vi "Modify_Power_ElectrodesDlg.vi"(6 "error in":errorcluster, 8 "一行记录":string[](array[string])) -> (0 "error out":errorcluster)   [LabVIEW 2014, in "PowerElectrodes.lvlib"]
uses:
  PowerElectrodes.lvlib
  DataBase/DataBase.lvlib
  DetectElecrodes/DetectElectros.lvlib
panel:
  out "结果字符串":string
  in  "继电器极性":enum16{"负", "正", "    "}(ring)
  out "区域名称":string
  in  "确定按钮":bool
  in  "取消按钮":bool
  in  "继电器名称":string
  in  "电极描述":string
  in  "电极位置":string
  in  "坐标Z":string
  in  "坐标Y":string
  in  "坐标X":string
  in  "电极名称":string
  in  "区域名称":u16(ring) items=["1区", "2区"]
  in  "OK":bool
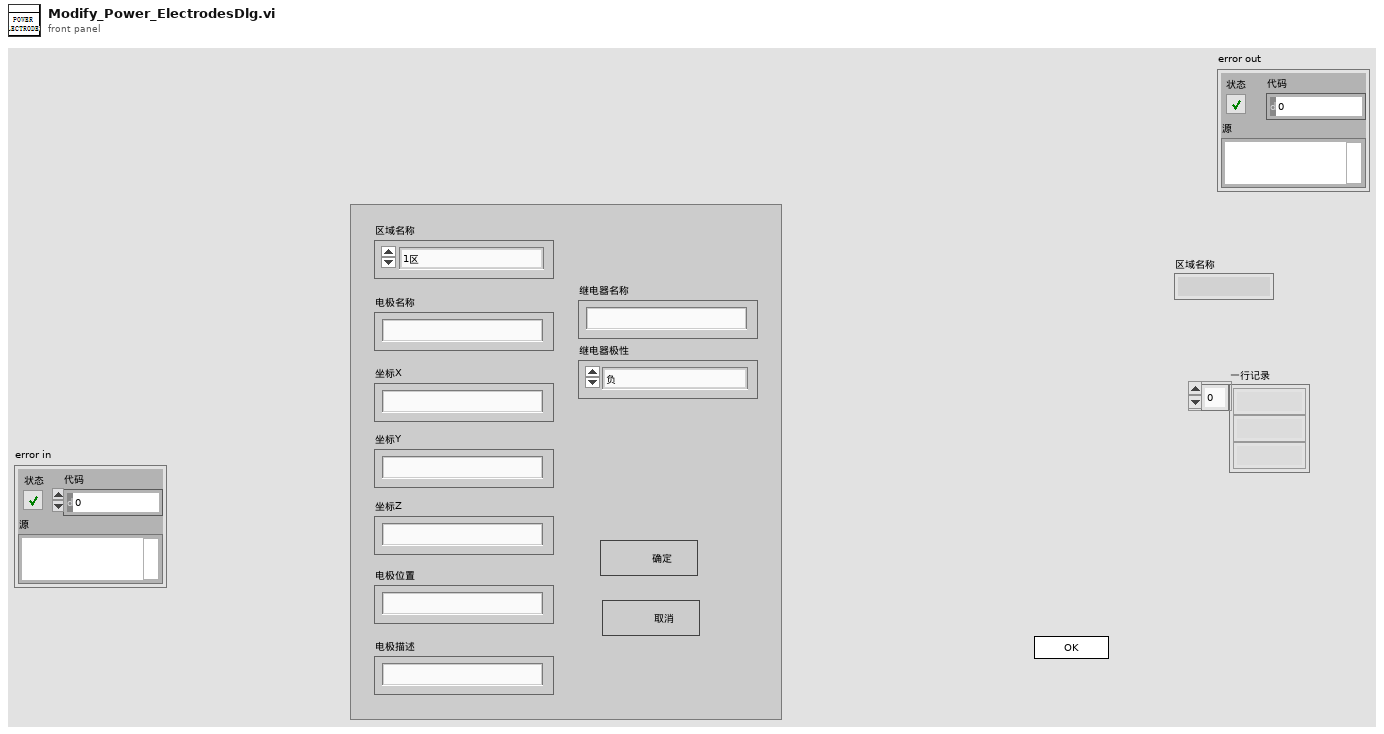
[diagram p1: front panel]
types:
  T1 = enum32{"invalid app kind", "Development System", "Run Time System", "Student Edition", "Embedded LabVIEW", "Evaluation", "Custom"}
  T2 = enum32{"Invalid", "Standard", "Closed", "Hidden", "Minimized", "Maximized"}
  T3 = cluster{"Core":cluster{"Current VI Reference":refnum<vi>, "Close Panel on Exit?":bool}, "Your Boolean data":bool, "Your string data":string, "AreaName":string[], "DataP":cluster{i32, "电极名称":string, "区域名称":string, "坐标X":string, "坐标Y":string, "坐标Z":string, "电极位置":string, "继电器名称":string, "继电器极性":string, "电极描述":string}, "一行记录D":string[], "power_id":string}
  T4 = cluster{i32, "电极名称":string, "区域名称":string, "坐标X":string, "坐标Y":string, "坐标Z":string, "电极位置":string, "继电器名称":string, "继电器极性":string, "电极描述":string}
  T5 = cluster{"Current VI Reference":refnum<vi>, "Close Panel on Exit?":bool}
  T6 = cluster{i32, "电极名称":string, "区域名称":string, "坐标X":string, "坐标Y":string, "坐标Z":string, "电极位置":string, "继电器名称":string, string, "电极描述":string}
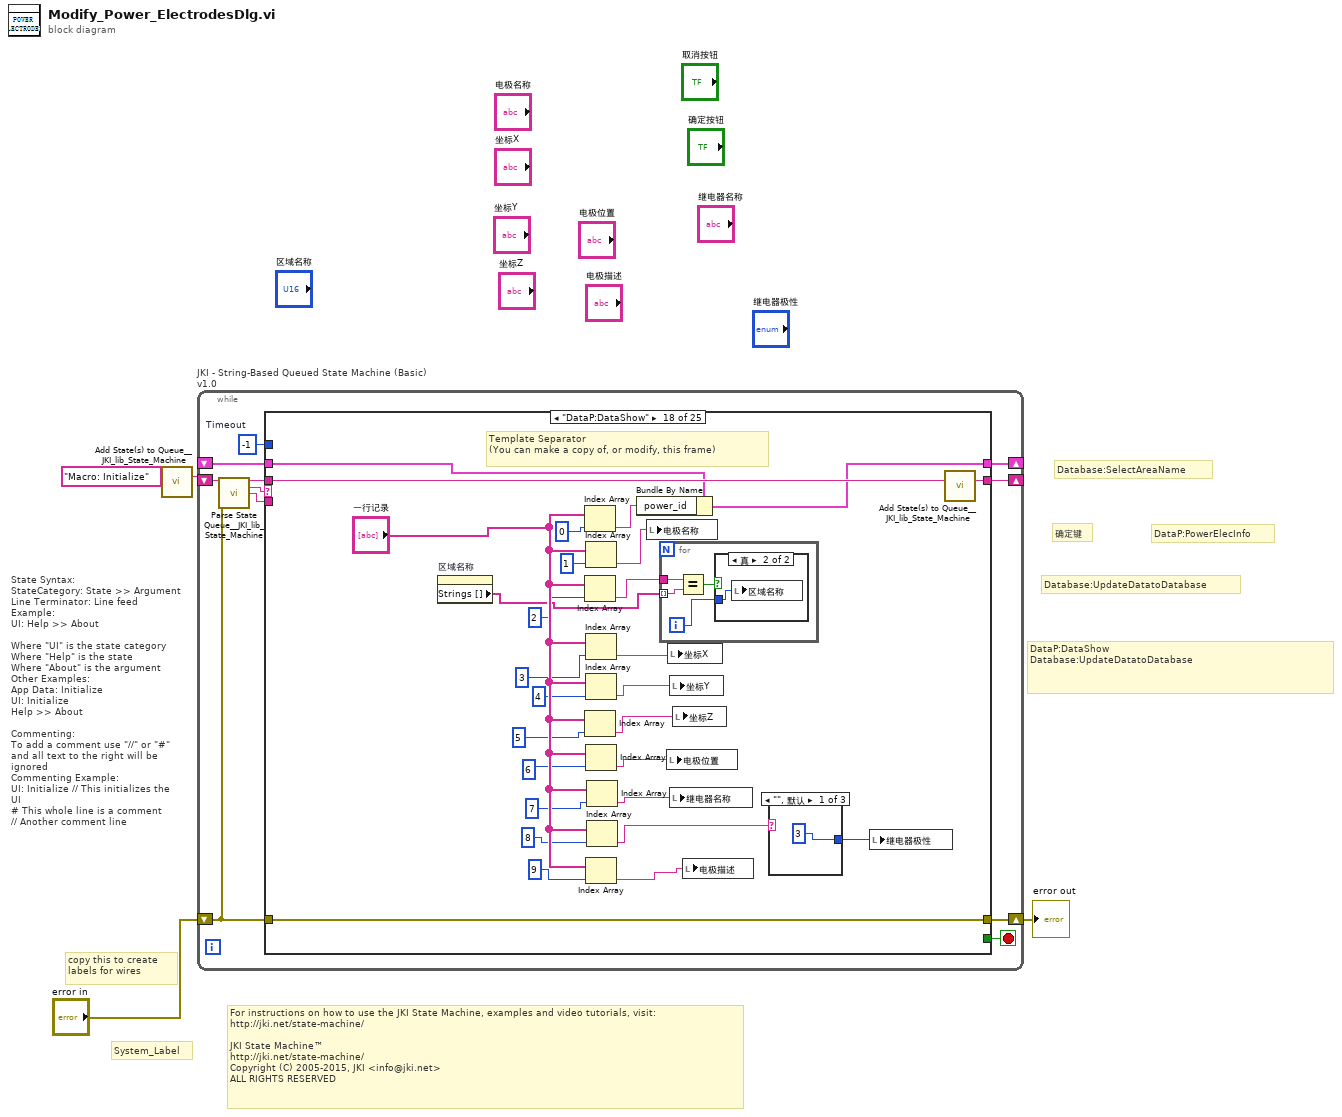
[diagram p0: block diagram]
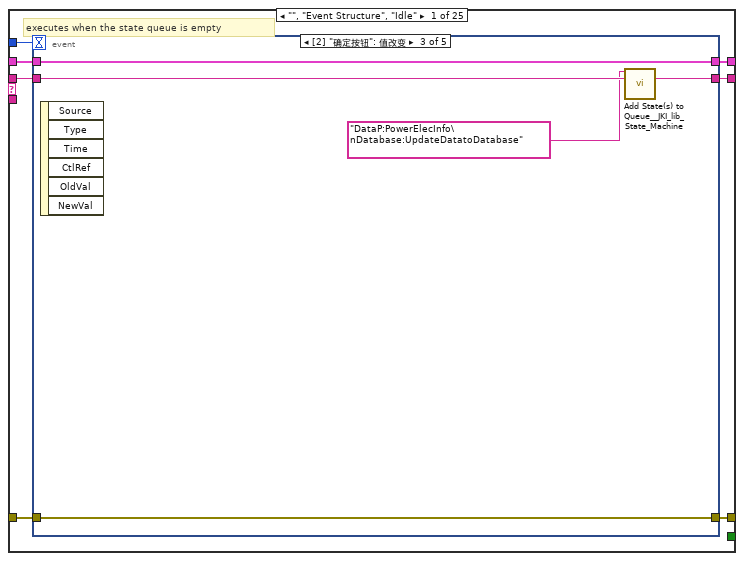
[diagram p2: hidden frame]
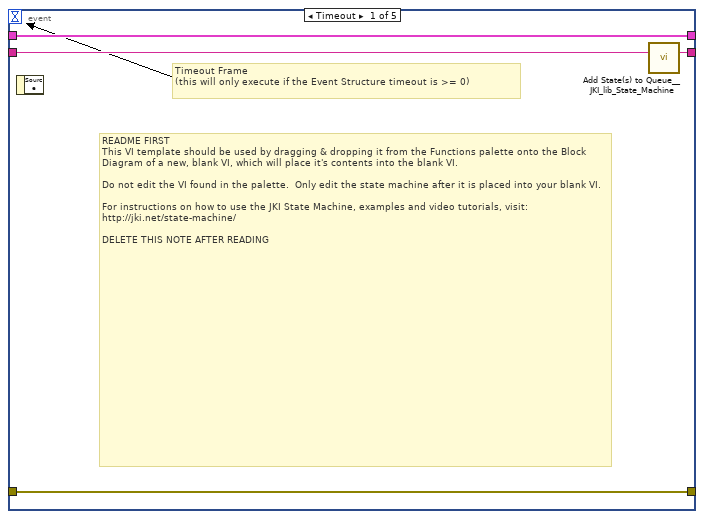
[diagram p3: hidden frame]
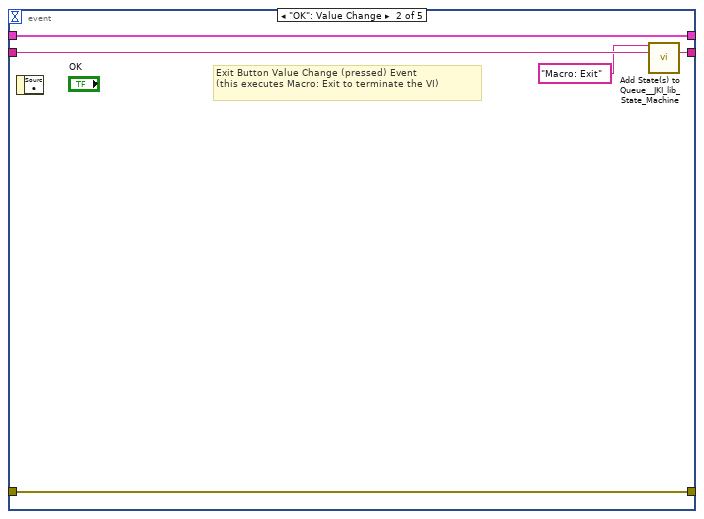
[diagram p4: hidden frame]
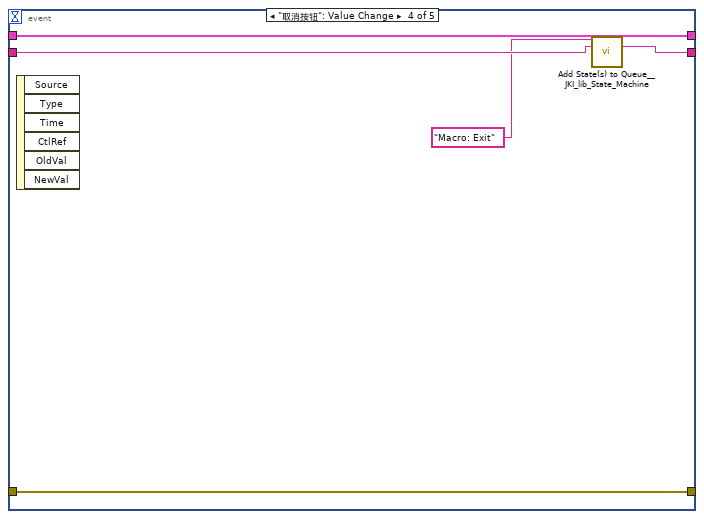
[diagram p5: hidden frame]
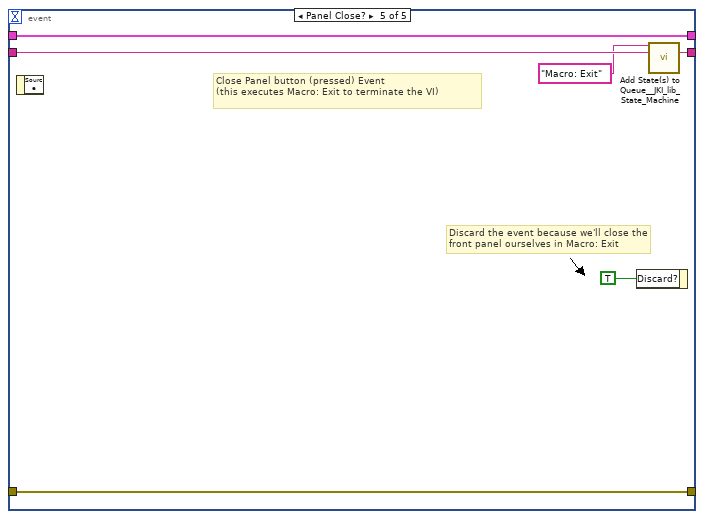
[diagram p6: hidden frame]
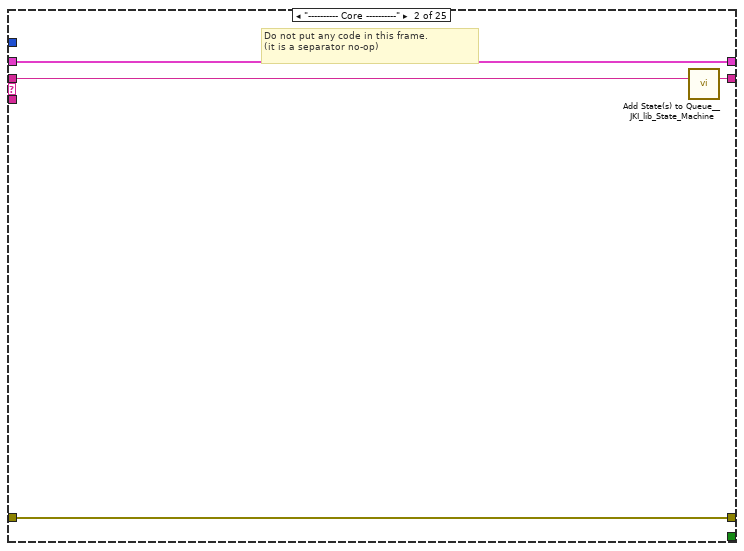
[diagram p7: hidden frame]
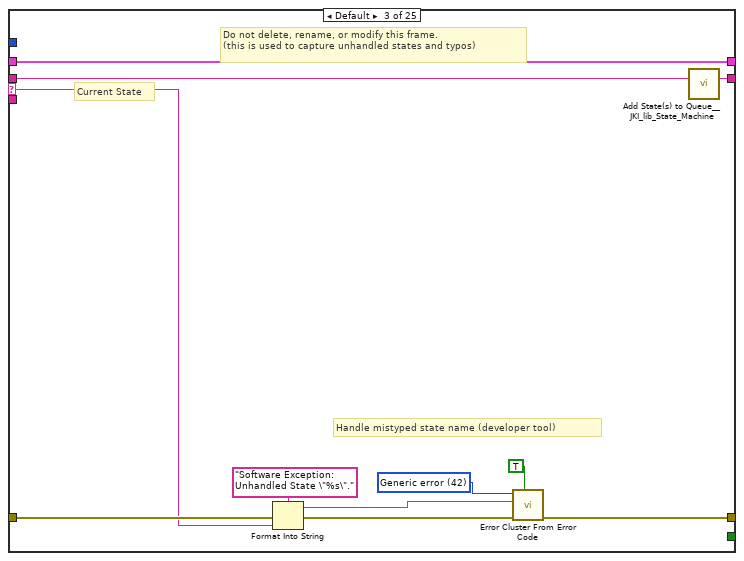
[diagram p8: hidden frame]
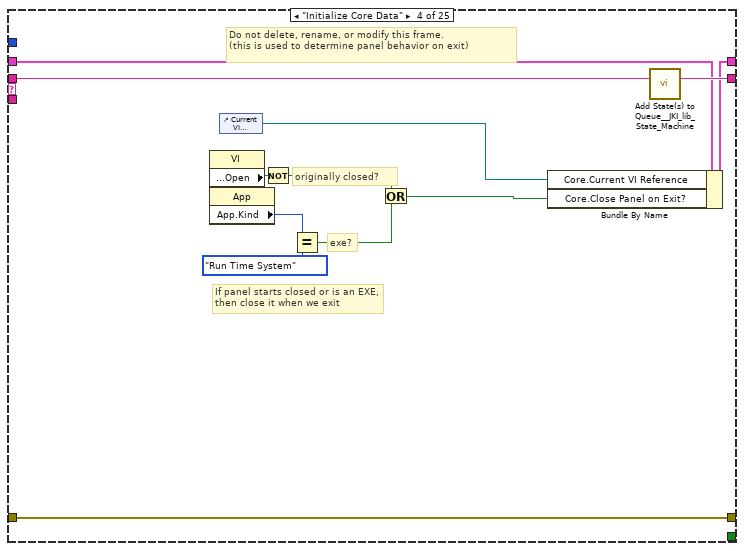
[diagram p9: hidden frame]
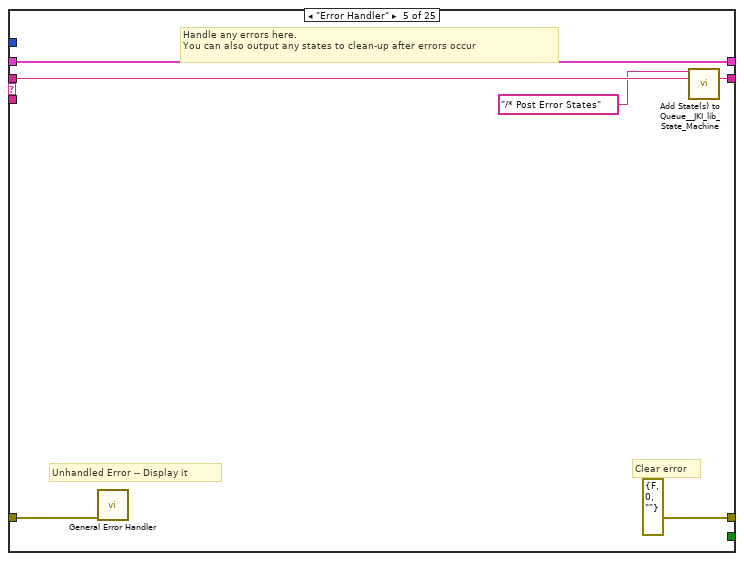
[diagram p10: hidden frame]
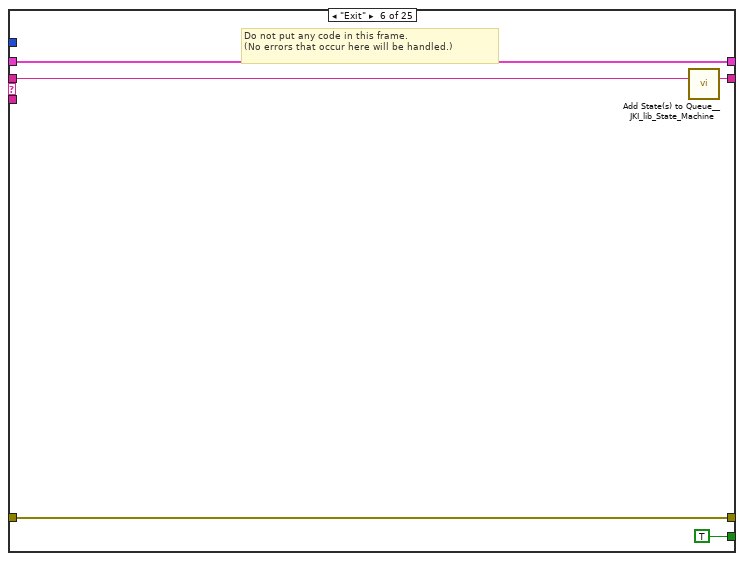
[diagram p11: hidden frame]
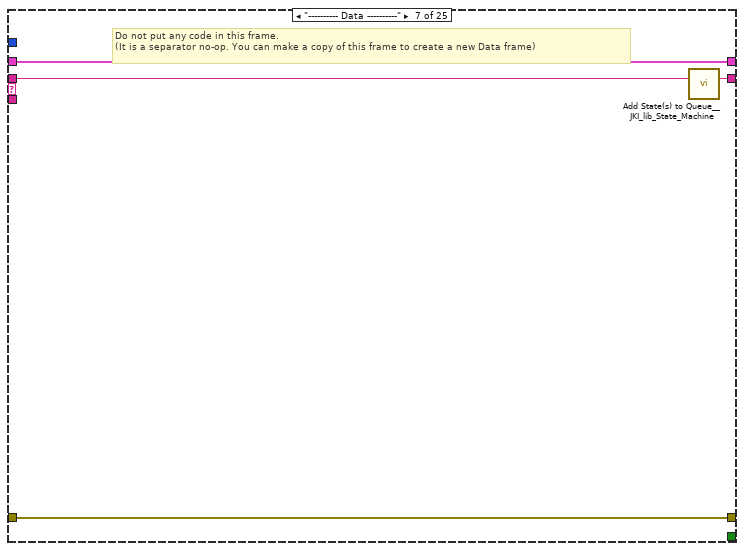
[diagram p12: hidden frame]
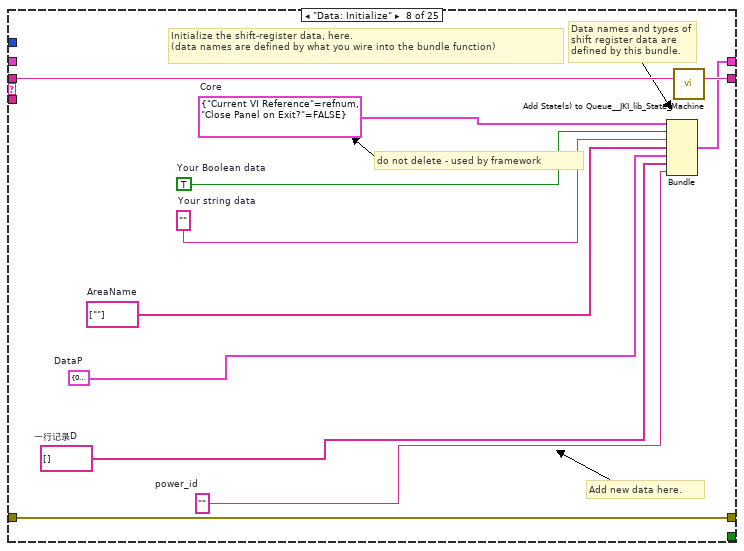
[diagram p13: hidden frame]
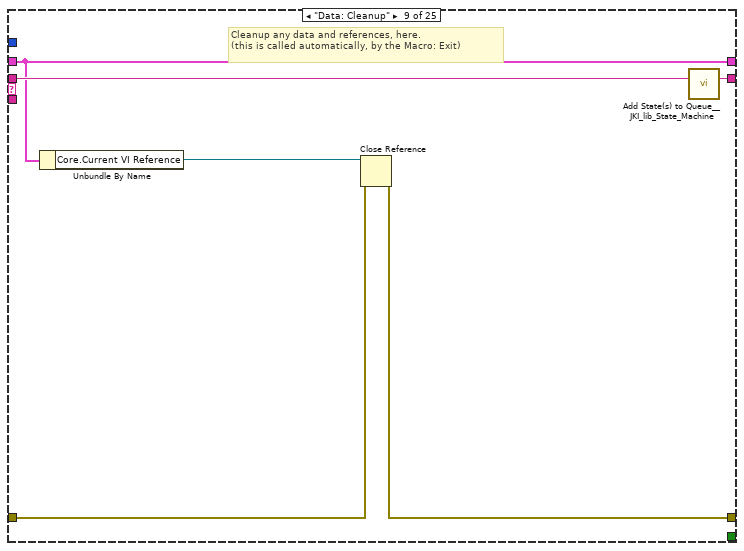
[diagram p14: hidden frame]
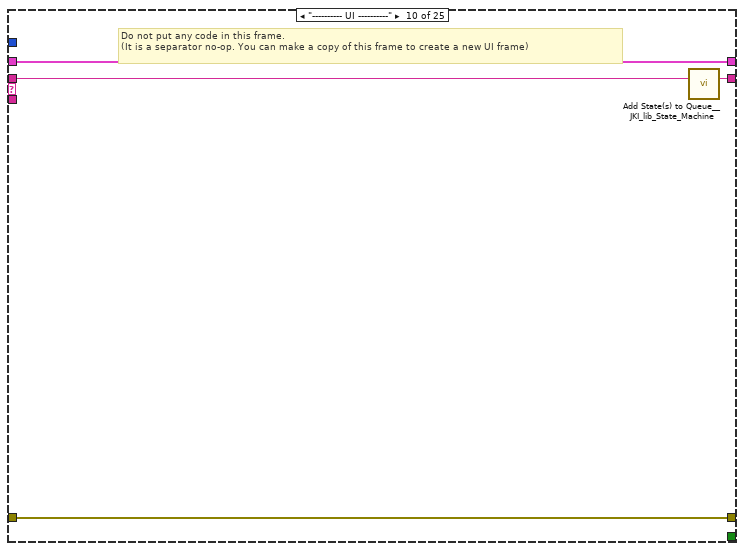
[diagram p15: hidden frame]
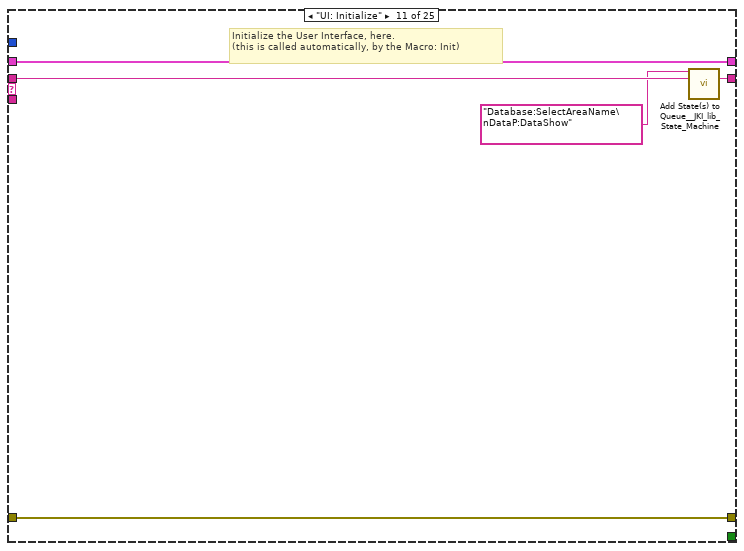
[diagram p16: hidden frame]
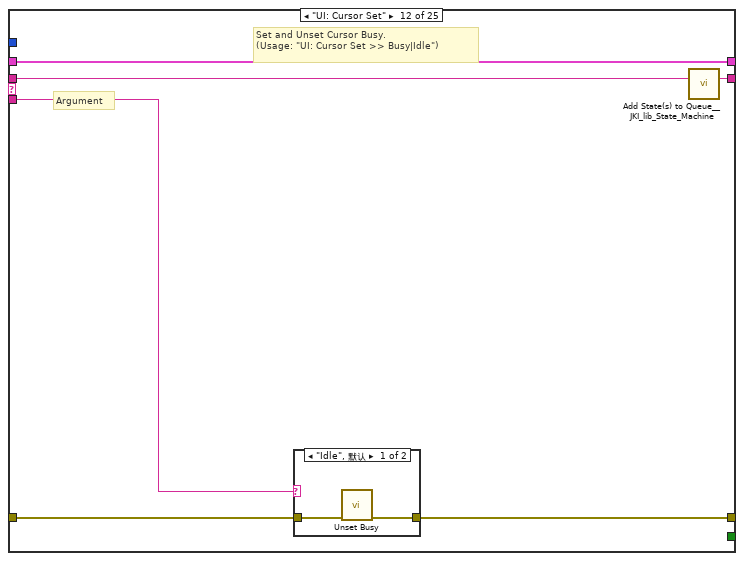
[diagram p17: hidden frame]
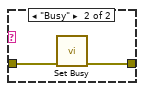
[diagram p18: hidden frame]
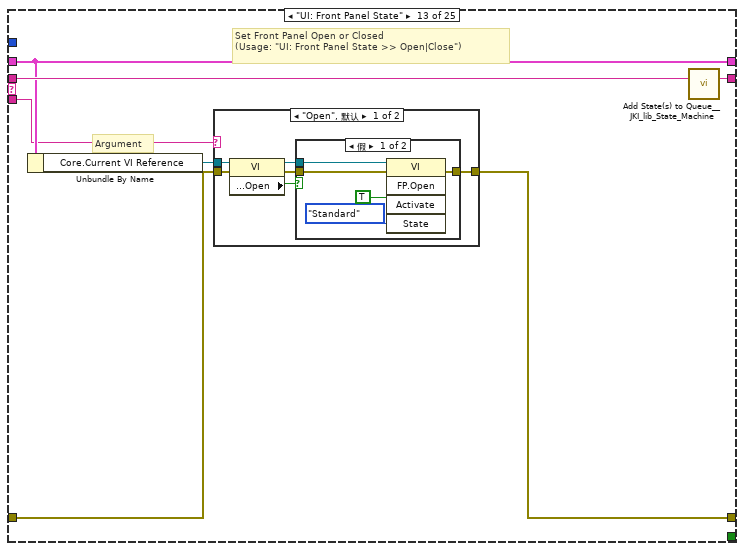
[diagram p19: hidden frame]
diagram:
  # "Database:UpdateDatatoDatabase"
  # "DataP:DataShow\nDatabase:UpdateDatatoDatabase"
  # "DataP:PowerElecInfo"
  # "确定键"
  # "Database:SelectAreaName"
  # "For instructions on how to use the JKI State Machine, examples and video tutorials, visit:\nhttp://jki.net/state-machine/\n\nJKI State Machine™\nhttp://jki.net/state-machine/\nCopyright (C) 2005-2015, JKI <info@jki.net>\nALL RIGHTS RESERVED"
  # "State Syntax:\nStateCategory: State >> Argument\nLine Terminator: Line feed\nExample:\nUI: Help >> About\n\nWhere \"UI\" is the state category\nWhere \"Help\" is the state\nWhere \"About\" is the argument\nOther Examples:\nApp Data: Initialize\nUI: Initialize\nHelp >> About\n\nCommenting:\nTo add a comment use \"//\" or \"#\" and all text to the right will be ignored\nCommenting Example:\nUI: Initialize // This initializes the UI\n# This whole line is a comment\n// Another comment line"
  # "copy this to create labels for wires"
  # "System_Label"
  n1 = call <vilib>:"Add State(s) to Queue__JKI_lib_State_Machine.vi"("State(s) in (\"\")"="Macro: Initialize") -> ("States Out"=w4:string)  [unwired: 14 in]
  n2 = while "JKI - String-Based Queued State Machine (Basic) v1.0" {
    shift-right: [w8] -> _
    shift-left: _ -> [w7]
    shift-right: [w11] -> w1
    shift-left: "error in" -> [w5]
    shift-right: [w10] -> _
    shift-left: w4 -> [w12]
    stop <- w9 stop-if-true
    w6 = -1  # Timeout
    n3 = call <vilib>:"Parse State Queue__JKI_lib_State_Machine.vi"("State Queue"=w12, "Error In (no error)"=w5) -> ("Remaining States"=w14:string, "Current State"=w15:string, "Arguments"=w13:string)  [unwired: 11 in]
    n4 = case shown="\"DataP:DataShow\"" w15 {
      selector: w15 -> [_ _ w52 _ _ _ _ _ _ _ _ _ _ _ _ _ _ _ _ _ _ _ _ _ _]
      tunnel: w14 -> [w22 w51 w56 w74 w80 w85 w89 w100 w106 w110 w115 w121 w132 w158 w163 w173 w177 w205 w234 w238 w260 w272 w276 w280 w284]
      tunnel: w13 -> [_ _ _ _ _ _ _ _ _ _ _ w116 w126 _ _ _ _ _ _ _ _ _ _ _ _]
      tunnel: w7 -> [w20 w48 w54 w65 w77 w83 w86 _ w101 w107 w113 w119 w128 w155 w160 w170 w174 w179 w220 w235 w257 w262 w273 w277 w281]
      tunnel: [w19 w49 w58 w71 errorcluster {"status"=FALSE, "code"=0, "source"=""} ("error out") w82 w87 w97 w102 w108 w111 w117 w129 w156 w161 w171 w175 w203 w232 w236 w240 w270 w274 w278 w282] -> w11
      tunnel: w5 -> [w18 w49 w57 w71 w76 w82 w87 w97 w103 w108 w111 w118 w130 w156 w161 w171 w175 w203 w232 w236 w239 w270 w274 w278 w282]
      tunnel: [w21 w50 w55 w73 w79 w84 w88 w99 w105 w109 w114 w120 w131 w157 w162 w172 w176 w204 w233 w237 w259 w271 w275 w279 w283] -> w10
      tunnel: [_ _ _ _ _ TRUE _ _ _ _ _ _ _ _ _ _ _ _ _ _ _ _ _ _ _] -> w9
      tunnel: [w17 w48 w54 w72 w77 w83 w86 w98 w101 w107 w113 w119 w128 w155 w160 w170 w174 w178 w219 w235 w257 w261 w273 w277 w281] -> w8
      tunnel: w6 -> [w16 _ _ _ _ _ _ _ _ _ _ _ _ _ _ _ _ _ _ _ _ _ _ _ _]
      frame "", "Event Structure", "Idle" {
        # "executes when the state queue is empty"
        n5 = event shown="[2] \"确定按钮\": 值改变" {
          selector: _ -> [_ _ _ _ _]
          dyn-events: _ -> [_ _ _ _ _]
          timeout: w16 -> [_ _ _ _ _]
          tunnel: w22 -> [w26 w31 w33 w39 w47]
          tunnel: [w25 w30 w34 w40 w46] -> w21
          tunnel: w20 -> [w23 w28 w36 w41 w44]
          tunnel: [w24 w29 w35 w37 w45] -> w19
          tunnel: w18 -> [w24 w29 w35 w37 w45]
          tunnel: [w23 w28 w36 w41 w44] -> w17
          event Timeout {
            # "README FIRST\nThis VI template should be used by dragging & dropping it from the Functions palette onto the Block Diagram of a new, blank VI, which will place it's contents into the blank VI.\n\nDo not edit the VI found in the palette.  Only edit the state machine after it is placed into your blank VI.\n\nFor instructions on how to use the JKI State Machine, examples and video tutorials, visit:\nhttp://jki.net/state-machine/\n\nDELETE THIS NOTE AFTER READING"
            # "Timeout Frame\n(this will only execute if the Event Structure timeout is >= 0)"
            n6 = event-data() -> ()  [unwired: 1 in, 1 out]
            n7 = call <vilib>:"Add State(s) to Queue__JKI_lib_State_Machine.vi"("State(s) in (\"\")"=w26) -> ("States Out"=w25:string)  [unwired: 14 in]
          }
          event "OK": Value Change {
            # "Exit Button Value Change (pressed) Event\n(this executes Macro: Exit to terminate the VI)"
            n8 = event-data() -> ()  [unwired: 1 in, 1 out]
            n9 = call <vilib>:"Add State(s) to Queue__JKI_lib_State_Machine.vi"("State(s) in Front (\"\")"="Macro: Exit", "State(s) in (\"\")"=w31) -> ("States Out"=w30:string)  [unwired: 13 in]
          }
          event "确定按钮": Value Change {
            n10 = event-data() -> ()  [unwired: 1 in, 6 out]
            n11 = call <vilib>:"Add State(s) to Queue__JKI_lib_State_Machine.vi"("State(s) in Front (\"\")"="DataP:PowerElecInfo\nDatabase:UpdateDatatoDatabase", "State(s) in (\"\")"=w33) -> ("States Out"=w34:string)  [unwired: 13 in]
          }
          event "取消按钮": Value Change {
            n12 = event-data() -> ()  [unwired: 1 in, 6 out]
            n13 = call <vilib>:"Add State(s) to Queue__JKI_lib_State_Machine.vi"("State(s) in Front (\"\")"="Macro: Exit", "State(s) in (\"\")"=w39) -> ("States Out"=w40:string)  [unwired: 13 in]
          }
          event Panel Close? {
            # "Discard the event because we'll close the front panel ourselves in Macro: Exit"
            # "Close Panel button (pressed) Event\n(this executes Macro: Exit to terminate the VI)"
            n14 = event-data() -> ()  [unwired: 1 in, 1 out]
            n15 = event-data("Discard?"=TRUE) -> ()  [unwired: 1 in, 1 out]
            n16 = call <vilib>:"Add State(s) to Queue__JKI_lib_State_Machine.vi"("State(s) in Front (\"\")"="Macro: Exit", "State(s) in (\"\")"=w47) -> ("States Out"=w46:string)  [unwired: 13 in]
          }
        }
      }
      frame "---------- Core ----------" {
        # "Do not put any code in this frame.\n(it is a separator no-op)"
        n17 = call <vilib>:"Add State(s) to Queue__JKI_lib_State_Machine.vi"("State(s) in (\"\")"=w51) -> ("States Out"=w50:string)  [unwired: 14 in]
      }
      frame Default {
        w61 = 42 items=["No error", "Argument error", "Memory is full", "Out of zone", "End of file", "File already open", "Generic file I/O error", "File not found", "File permission error", "Disk is full", "Duplicate path", "Too many files open", "System feature not enabled", "Resource file not found", "Cannot add resource", "Resource not found", "Image not found", "Image memory error", "Pen does not exist", "Config type invalid", "Config token not found", "Config parse error", "Config memory error", "Bad external code format", "Bad external code offset", "External code not present", "Null window", "Destroy window error", "Null menu", "Print aborted", "Bad print record", "Print driver error", "Windows error during printing", "Memory error during printing", "Print dialog error", "Generic print error", "Invalid device refnum", "Device not found", "Device parameter error", "Device unit error", "Cannot open device", "Device call aborted", "Generic error", "Cancelled by user", "Object ID too low", "Object ID too high", "Object not in heap", "Unknown heap", "Unknown object (invalid DefProc)", "Unknown object (DefProc not in table)", "Message out of range", "Invalid (null) method", "Unknown message", "Manager call not supported", "Bad address", "Network operation in progress", "Network operation timed out", "Connection is busy", "Network attribute not supported", "Network error", "Address in use", "System out of memory", "Connection aborted", "Connection refused", "Not connected", "Already connected", "Connection closed", "Initialization error (interapplication manager)", "Bad occurrence", "Wait on unbound occurrence handler", "Occurrence queue overflow", "Datalog type conflict", "Unused", "Unrecognized type (interapplication manager)", "Memory corrupt", "Failed to make temporary DLL", "Old CIN version", "Drag socket not found", "Failed to load drop-object", "Failed to register OLE object", "Failed to release OLE object", "Format specifier type mismatch", "Unknown format specifier", "Too few format specifiers", "Too many format specifiers", "Scan failed", "Newer CIN version", "Error converting to variant", "Runtime menu error", "Password tampered", "Variant attribute not found", "Incompatible variant data type", "Event data is not available", "Event Store is not present", "Occurrence is not found", "Event Queue is not created", "Event info is not available", "Refnum passed is NULL", "Error retrieving Class GUID", "Error retrieving CoClass GUID", "Error retrieving TypeLib GUID.", "Bad built application magic bytes.", "Specific driver is different from the specific driver associated with the Logical Name.", "There is no session opened to the class driver.", "Max Error", "MAX - Error with config objects", "MAX - Error loading configuration", "MAX - Group not supported"]
        # "Current State"
        # "Do not delete, rename, or modify this frame.\n(this is used to capture unhandled states and typos)"
        # "Handle mistyped state name (developer tool)"
        n18 = Format Into String(format string="Software Exception: Unhandled State \"%s\"." ("message"), error in=w57, w52) -> (resulting string=w60:string, error out=w59:errorcluster)  [unwired: 1 in]
        n19 = call <vilib>:"Error Cluster From Error Code.vi"("show call chain? (False)"=TRUE, "error in (no error)"=w59, "error message (\"\")"=w60, "error code (0)"=w61) -> ("error out"=w58:errorcluster)  [unwired: 5 in]
        n20 = call <vilib>:"Add State(s) to Queue__JKI_lib_State_Machine.vi"("State(s) in (\"\")"=w56) -> ("States Out"=w55:string)  [unwired: 14 in]
      }
      frame "Initialize Core Data" {
        # "Do not delete, rename, or modify this frame.\n(this is used to determine panel behavior on exit)"
        # "originally closed?"
        # "exe?"
        # "If panel starts closed or is an EXE, then close it when we exit"
        n21 = property class="VI"() -> ("Front Panel.Open"=w70:bool)  [unwired: 2 in, 2 out]
        n22 = property class="App"() -> ("App.Kind"=w69:T1)  [unwired: 2 in, 2 out]
        n23 = control-ref of="Current VI Reference"() -> (w63:refnum<vi>)
        n24 = Not(x=w70) -> (.not. x?=w67:bool)
        n25 = Equal?(x=w69, y=T1."Run Time System" ("Application:Kind")) -> (x = y?=w66:bool)
        n26 = Or(x=w67, y=w66) -> (x .or. y?=w64:bool)
        n27 = Bundle By Name(cluster=w65, "Core.Current VI Reference"=w63, "Core.Close Panel on Exit?"=w64) -> (w72:T3)
        n28 = call <vilib>:"Add State(s) to Queue__JKI_lib_State_Machine.vi"("State(s) in (\"\")"=w74) -> ("States Out"=w73:string)  [unwired: 14 in]
      }
      frame "Error Handler" {
        # "Unhandled Error -- Display it"
        # "Handle any errors here.\nYou can also output any states to clean-up after errors occur"
        # "Clear error"
        n29 = call <vilib>:"General Error Handler.vi"("error in (no error)"=w76) -> ()  [unwired: 10 in, 5 out]
        n30 = call <vilib>:"Add State(s) to Queue__JKI_lib_State_Machine.vi"("State(s) in Front (\"\")"="/* Post Error States", "State(s) in (\"\")"=w80) -> ("States Out"=w79:string)  [unwired: 13 in]
      }
      frame "Exit" {
        # "Do not put any code in this frame.\n(No errors that occur here will be handled.)"
        n31 = call <vilib>:"Add State(s) to Queue__JKI_lib_State_Machine.vi"("State(s) in (\"\")"=w85) -> ("States Out"=w84:string)  [unwired: 14 in]
      }
      frame "---------- Data ----------" {
        # "Do not put any code in this frame.\n(It is a separator no-op. You can make a copy of this frame to create a new Data frame)"
        n32 = call <vilib>:"Add State(s) to Queue__JKI_lib_State_Machine.vi"("State(s) in (\"\")"=w89) -> ("States Out"=w88:string)  [unwired: 14 in]
      }
      frame "Data: Initialize" {
        w90 = ""  # power_id
        w91 = string[] []  # 一行记录D
        w92 = T4 {0, "电极名称"="", "区域名称"="", "坐标X"="", "坐标Y"="", "坐标Z"="", "电极位置"="", "继电器名称"="", "继电器极性"="", "电极描述"=""}  # DataP
        w93 = string[] [""]  # AreaName
        w94 = T5 {"Current VI Reference"=refnum, "Close Panel on Exit?"=FALSE}  # Core
        w96 = TRUE  # Your Boolean data
        w95 = ""  # Your string data
        # "do not delete - used by framework"
        # "Add new data here."
        # "Data names and types of shift register data are defined by this bundle."
        # "Initialize the shift-register data, here.\n(data names are defined by what you wire into the bundle function)"
        n33 = Bundle("Core"=w94, "Your Boolean data"=w96, "Your string data"=w95, "AreaName"=w93, "DataP"=w92, "一行记录D"=w91, "power_id"=w90) -> (w98:T3)  [unwired: 1 in]
        n34 = call <vilib>:"Add State(s) to Queue__JKI_lib_State_Machine.vi"("State(s) in (\"\")"=w100) -> ("States Out"=w99:string)  [unwired: 14 in]
      }
      frame "Data: Cleanup" {
        # "Cleanup any data and references, here.\n(this is called automatically, by the Macro: Exit)"
        n35 = Unbundle By Name(w101) -> ("Core.Current VI Reference"=w104:refnum<vi>)
        n36 = Close Reference(reference=w104, error in (no error)=w103) -> (error out=w102:errorcluster)
        n37 = call <vilib>:"Add State(s) to Queue__JKI_lib_State_Machine.vi"("State(s) in (\"\")"=w106) -> ("States Out"=w105:string)  [unwired: 14 in]
      }
      frame "---------- UI ----------" {
        # "Do not put any code in this frame.\n(It is a separator no-op. You can make a copy of this frame to create a new UI frame)"
        n38 = call <vilib>:"Add State(s) to Queue__JKI_lib_State_Machine.vi"("State(s) in (\"\")"=w110) -> ("States Out"=w109:string)  [unwired: 14 in]
      }
      frame "UI: Initialize" {
        # "Initialize the User Interface, here.\n(this is called automatically, by the Macro: Init)"
        n39 = call <vilib>:"Add State(s) to Queue__JKI_lib_State_Machine.vi"("State(s) in Front (\"\")"="Database:SelectAreaName\nDataP:DataShow", "State(s) in (\"\")"=w115) -> ("States Out"=w114:string)  [unwired: 13 in]
      }
      frame "UI: Cursor Set" {
        # "Argument"
        # "Set and Unset Cursor Busy.\n(Usage: \"UI: Cursor Set >> Busy|Idle\")"
        n40 = case shown="\"Idle\", 默认" w116 {
          tunnel: w118 -> [w123 w125]
          tunnel: [w122 w124] -> w117
          frame "Idle", Default {
            n41 = call <vilib>:"Unset Busy.vi"("error in (no error)"=w123) -> ("error out"=w122:errorcluster)  [unwired: 10 in]
          }
          frame "Busy" {
            n42 = call <vilib>:"Set Busy.vi"("error in (no error)"=w125) -> ("error out"=w124:errorcluster)  [unwired: 9 in, 1 out]
          }
        }
        n43 = call <vilib>:"Add State(s) to Queue__JKI_lib_State_Machine.vi"("State(s) in (\"\")"=w121) -> ("States Out"=w120:string)  [unwired: 14 in]
      }
      frame "UI: Front Panel State" {
        # "Argument"
        # "Set Front Panel Open or Closed\n(Usage: \"UI: Front Panel State >> Open|Close\")"
        n44 = Unbundle By Name(w128) -> ("Core.Current VI Reference"=w127:refnum<vi>)
        n45 = case shown="\"Open\", 默认" w126 {
          tunnel: w130 -> [w136 w149]
          tunnel: [w138 w150] -> w129
          tunnel: w127 -> [w137 w147]
          frame "Open", Default {
            n46 = property class="VI"(reference=w137, error in=w136) -> (reference out=w134:refnum<vi>, error out=w135:errorcluster, "Front Panel.Open"=w133:bool)
            n47 = case shown="假" w133 {
              tunnel: [w141 w144] -> w138
              tunnel: w135 -> [w140 w144]
              tunnel: w134 -> [w139 _]
              frame False {
                n48 = invoke class="VI" method="FP.Open"(reference=w139, error in=w140, "Activate"=TRUE, "State"=T2."Standard") -> (error out=w141:errorcluster)  [unwired: 1 in, 4 out]
              }
              frame True {
              }
            }
          }
          frame "Close" {
            n49 = property class="VI"(reference=w147, error in=w149) -> (reference out=w146:refnum<vi>, error out=w148:errorcluster, "Front Panel.Open"=w145:bool)
            n50 = case shown="真" w145 {
              tunnel: [w151 w154] -> w150
              tunnel: w148 -> [w151 w153]
              tunnel: w146 -> [_ w152]
              frame False {
              }
              frame True {
                n51 = invoke class="VI" method="FP.Close"(reference=w152, error in=w153) -> (error out=w154:errorcluster)  [unwired: 1 in, 2 out]
              }
            }
          }
        }
        n52 = call <vilib>:"Add State(s) to Queue__JKI_lib_State_Machine.vi"("State(s) in (\"\")"=w132) -> ("States Out"=w131:string)  [unwired: 14 in]
      }
      frame "---------- Macro ----------" {
        # "Do not put any code in this frame.\n(It is a separator no-op. You can make a copy of this frame to create a new Macro frame)"
        n53 = call <vilib>:"Add State(s) to Queue__JKI_lib_State_Machine.vi"("State(s) in (\"\")"=w158) -> ("States Out"=w157:string)  [unwired: 14 in]
      }
      frame "Macro: Initialize" {
        w159 = "Data: Initialize\nInitialize Core Data\nUI: Initialize\nUI: Front Panel State >> Open"  # Data: Initialize Initialize Core Data UI: Initialize UI: Front Panel State >> Open
        # "Initialization Macro\n(This is called once, when the VI starts)"
        n54 = call <vilib>:"Add State(s) to Queue__JKI_lib_State_Machine.vi"("State(s) in Front (\"\")"=w159, "State(s) in (\"\")"=w163) -> ("States Out"=w162:string)  [unwired: 13 in]
      }
      frame "Macro: Exit" {
        # "Exit Macro\n(This is called once, when the VI exits)"
        n55 = Unbundle By Name(w170) -> ("Core.Close Panel on Exit?"=w169:bool)
        n56 = Select(t="UI: Front Panel State >> Close", s=w169, f="") -> (s? t:f=w166:string)
        n57 = call <vilib>:"Add State(s) to Queue__JKI_lib_State_Machine.vi"("State(s) in (\"\")"=w166, "State(s) at Back (\"\")"="Data: Cleanup\nExit") -> ("States Out"=w164:string)  [unwired: 13 in]
        n58 = call <vilib>:"Add State(s) to Queue__JKI_lib_State_Machine.vi"("State(s) in Front (\"\")"=w164, "State(s) in (\"\")"=w173) -> ("States Out"=w172:string)  [unwired: 13 in]
      }
      frame "-----------DataP-----------" {
        # "Template Separator\n(You can make a copy of, or modify, this frame)"
        n59 = call <vilib>:"Add State(s) to Queue__JKI_lib_State_Machine.vi"("State(s) in (\"\")"=w177) -> ("States Out"=w176:string)  [unwired: 14 in]
      }
      frame "DataP:DataShow" {
        # "Template Separator\n(You can make a copy of, or modify, this frame)"
        n60 = property on="区域名称" class="Ring (严格)"() -> ("Strings []"=w182:string[])  [unwired: 2 in, 2 out]
        n61 = Index Array(array="一行记录", index=0) -> (element=w180:string)
        n62 = Index Array(array="一行记录", index=2) -> (element=w181:string)
        n63 = Index Array(array="一行记录", index=5) -> (element=w188:string)
        n64 = Index Array(array="一行记录", index=1) -> (element=w191:string)
        n65 = Index Array(array="一行记录", index=3) -> (element=w190:string)
        n66 = Index Array(array="一行记录", index=4) -> (element=w189:string)
        n67 = Index Array(array="一行记录", index=6) -> (element=w187:string)
        n68 = Index Array(array="一行记录", index=9) -> (element=w186:string)
        n69 = Index Array(array="一行记录", index=7) -> (element=w185:string)
        n70 = Index Array(array="一行记录", index=8) -> (element=w184:string)
        n71 = Bundle By Name(cluster=w179, "power_id"=w180) -> (w178:T3)
        n72 = local write "电极名称"(w191) -> ()
        n73 = for {
          tunnel: w182 -> [w209] mode=indexing
          tunnel: w181 -> [w208]
          i -> [w206]
          n74 = Equal?(x=w208, y=w209) -> (x = y?=w207:bool)
          n75 = case shown="真" w207 {
            tunnel: w206 -> [_ w210]
            frame False {
            }
            frame True {
              n76 = local write "区域名称"(w210) -> ()
            }
          }
        }
        n77 = local write "电极位置"(w187) -> ()
        n78 = local write "坐标X"(w190) -> ()
        n79 = local write "坐标Y"(w189) -> ()
        n80 = local write "继电器名称"(w185) -> ()
        n81 = local write "坐标Z"(w188) -> ()
        n82 = local write "电极描述"(w186) -> ()
        n83 = case shown="\"\", 默认" w184 {
          tunnel: [3 1 0] -> w183
          frame "", Default {
          }
          frame "正" {
          }
          frame "负" {
          }
        }
        n84 = local write "继电器极性"(w183) -> ()
        n85 = call <vilib>:"Add State(s) to Queue__JKI_lib_State_Machine.vi"("State(s) in (\"\")"=w205) -> ("States Out"=w204:string)  [unwired: 14 in]
      }
      frame "DataP:PowerElecInfo" {
        # "Template Separator\n(You can make a copy of, or modify, this frame)"
        n86 = local read "电极名称"() -> (w228:string)
        n87 = local read "电极位置"() -> (w224:string)
        n88 = local read "坐标Z"() -> (w225:string)
        n89 = local read "坐标Y"() -> (w226:string)
        n90 = local read "坐标X"() -> (w227:string)
        n91 = local read "区域名称"() -> (w230:u16)
        n92 = Unbundle By Name(w220) -> ("AreaName"=w231:string[])
        n93 = local read "区域名称"() -> (w218:string)
        n94 = local read "继电器名称"() -> (w223:string)
        n95 = Index Array(array=w231, index=w230) -> (element=→"区域名称":string)
        n96 = local read "电极描述"() -> (w222:string)
        n97 = local read "继电器极性"() -> (w215:enum16{"负", "正", "    "})
        n98 = Index Array(array=string[] ["负", "正", " "], index=w215) -> (element=w214:string)
        n99 = Bundle(0, "电极名称"=w228, "区域名称"=w218, "坐标X"=w227, "坐标Y"=w226, "坐标Z"=w225, "电极位置"=w224, "继电器名称"=w223, w214, "电极描述"=w222) -> (w221:T6)  [unwired: 1 in]
        n100 = Bundle By Name(cluster=w220, "DataP"=w221) -> (w219:T3)
        n101 = call <vilib>:"Add State(s) to Queue__JKI_lib_State_Machine.vi"("State(s) in (\"\")"=w234) -> ("States Out"=w233:string)  [unwired: 14 in]
      }
      frame "--------DataBase----------" {
        # "Your code here.\n(You can make a copy of, or modify, this frame)"
        n102 = call <vilib>:"Add State(s) to Queue__JKI_lib_State_Machine.vi"("State(s) in (\"\")"=w238) -> ("States Out"=w237:string)  [unwired: 14 in]
      }
      frame "Database:UpdateDatatoDatabase" {
        # "Your code here.\n(You can make a copy of, or modify, this frame)"
        n103 = Unbundle By Name(w257) -> ("power_id"=w245:string)
        n104 = local read "继电器名称"() -> (w250:string)
        n105 = local read "电极位置"() -> (w251:string)
        n106 = local read "电极名称"() -> (w255:string)
        n107 = local read "坐标Y"() -> (w253:string)
        n108 = local read "坐标X"() -> (w254:string)
        n109 = local read "坐标Z"() -> (w252:string)
        n110 = local read "电极描述"() -> (w246:string)
        n111 = local read "区域名称"() -> (w243:u16)
        n112 = property on="区域名称" class="Ring (严格)"() -> ("Strings []"=w244:string[])  [unwired: 2 in, 2 out]
        n113 = local read "继电器极性"() -> (w248:enum16{"负", "正", "    "})
        n114 = Index Array(array=w244, index=w243) -> (element=w242:string)
        n115 = Index Array(array=string[] ["负", "正", ""], index=w248) -> (element=w247:string)
        n116 = Format Into String(format string="update t_power_electrodes set\npower_electrodes_name='%s',\narea_name='%s',\npower_electrodes_gps_x='%s',\npower_electrodes_gps_y='%s',\npower_electrodes_gps_z='%s',\npower_electrodes_position='%s',\ndelay_name='%s',\ndelay_polarity='%s',\npower_electrodes_desc='%s' where\npower_electrodes_id='%s';", w255, w242, w254, w253, w252, w251, w250, w247, w246, w245) -> (resulting string=w241:string)  [unwired: 2 in, 1 out]
        "结果字符串" <- w241
        n117 = call "updateData.vi"("error in"=w239, "SQL query"=w241) -> ("error out"=w240:errorcluster)  [unwired: 9 in]
        n118 = call <vilib>:"Add State(s) to Queue__JKI_lib_State_Machine.vi"("State(s) in Front (\"\")"="Macro: Exit", "State(s) in (\"\")"=w260) -> ("States Out"=w259:string)  [unwired: 13 in]
      }
      frame "Database:SelectAreaName" {
        # "Your code here.\n(You can make a copy of, or modify, this frame)"
        n119 = call "SelectData.vi"("SQL query"="select  area_name from t_area;") -> ("recordset data"=w268:variant[][])  [unwired: 7 in, 1 out]
        n120 = call "ReadDataFromDatabase.vi"("长度"=1, "index"=0, "recordset data"=w268) -> ("所有记录"=w265:string[][])  [unwired: 7 in, 1 out]
        n121 = Index Array(array=w265, index (col)=0) -> (element=w263:string[])  [unwired: 1 in]
        n122 = property on="区域名称" class="Ring (严格)"("Strings []"=w263) -> ()  [unwired: 2 in, 2 out]
        n123 = Bundle By Name(cluster=w262, "AreaName"=w263) -> (w261:T3)
        n124 = call <vilib>:"Add State(s) to Queue__JKI_lib_State_Machine.vi"("State(s) in (\"\")"=w272) -> ("States Out"=w271:string)  [unwired: 14 in]
      }
      frame "---------- New Category ----------" {
        # "Template Separator\n(You can make a copy of, or modify, this frame)"
        n125 = call <vilib>:"Add State(s) to Queue__JKI_lib_State_Machine.vi"("State(s) in (\"\")"=w276) -> ("States Out"=w275:string)  [unwired: 14 in]
      }
      frame "New Category: 1" {
        # "Your code here.\n(You can make a copy of, or modify, this frame)"
        n126 = call <vilib>:"Add State(s) to Queue__JKI_lib_State_Machine.vi"("State(s) in (\"\")"=w280) -> ("States Out"=w279:string)  [unwired: 14 in]
      }
      frame "New Category: 2" {
        # "Your code here.\n(You can make a copy of, or modify, this frame)"
        n127 = call <vilib>:"Add State(s) to Queue__JKI_lib_State_Machine.vi"("State(s) in (\"\")"=w284) -> ("States Out"=w283:string)  [unwired: 14 in]
      }
    }
  }
  "error out" <- w1
